vi "Send Drone MAVLink Message.vi"(8 "error in (no error)":errorcluster, 11 "MAVLink Message":u8[](array[numeric])) -> (0 "error out":errorcluster)   [LabVIEW 2014]
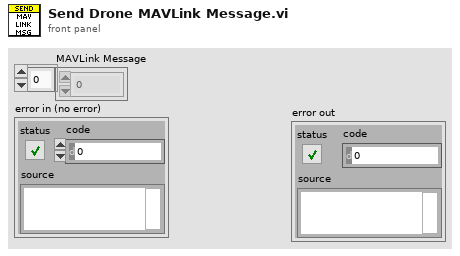
[diagram p1: front panel]
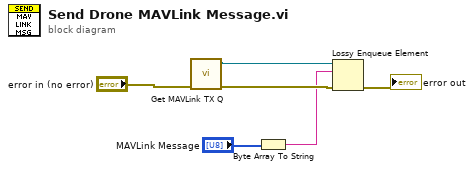
[diagram p0: block diagram]
diagram:
  n1 = call "Get MAVLink TX Q.vi"("error in (no error)"="error in (no error)") -> ("error out"=w5:errorcluster, "MAVLink Q"=w6:refnum<queue>)  [unwired: 9 in]
  n2 = Byte Array To String(unsigned byte array="MAVLink Message") -> (string=w3:string)
  n3 = Lossy Enqueue Element(queue=w6, element=w3, error in (no error)=w5) -> (error out=→"error out":errorcluster)  [unwired: 3 out]
